vi "Get Core Type.vi"(8 "error in (no error)":errorcluster, 11 "Multi Instrument Handler in":refnum<class "Multi Instrument Handler.lvclass">) -> (0 "error out":errorcluster, 3 "Sequencer Core out":refnum<class "Sequencer Core.lvclass">)   [LabVIEW 2020, in "Instrument Handler.lvlib" / "Multi Instrument Handler.lvclass"]
doc: "Return the Sequencer Core type to launch with the Sequencer.\n\nThis implementation returns the 'Multi Instrument Sequencer'."
uses:
  Multi Instrument Handler.lvclass
  PPL/HDH.Actor Framework.Core.Sequencer.lvlibp/Sequencer Core/Sequencer Core.lvclass
  Multi Instrument Sequencer/Multi Instrument Sequencer.lvclass
  C:/Current projects/WS/PPL/HDH.Actor Framework.Core.Sequencer.lvlibp/Sequencer Core/Sequencer Core.lvclass
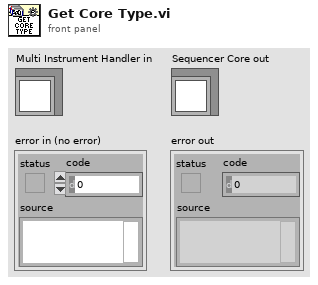
[diagram p1: front panel]
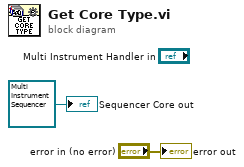
[diagram p0: block diagram]
diagram:
  "error out" <- "error in (no error)"
  "Sequencer Core out" <- refnum<class "Multi Instrument Sequencer.lvclass"> refnum ("Instrument Handler.lvlib:Multi Instrument Sequencer.lvclass")
